vi "FileIO.vi"() -> ()   [LabVIEW 2012]
uses:
  <vilib>/Utility/file.llb/Write To Spreadsheet File (string).vi
  <vilib>/Utility/file.llb/Write To Spreadsheet File (DBL).vi
  <vilib>/Utility/file.llb/Read From Spreadsheet File (DBL).vi
panel:
  out "spreadsheet path":path
  out "Result":dbl[][](array[numeric]) format="%0.3f"
  out "Result":string
  out "text path":path
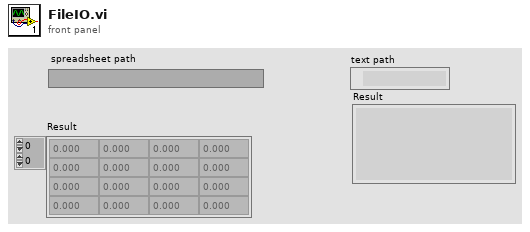
[diagram p1: front panel]
types:
  T1 = enum16{"open", "replace", "create", "open or create", "replace or create", "replace or create with confirmation"}
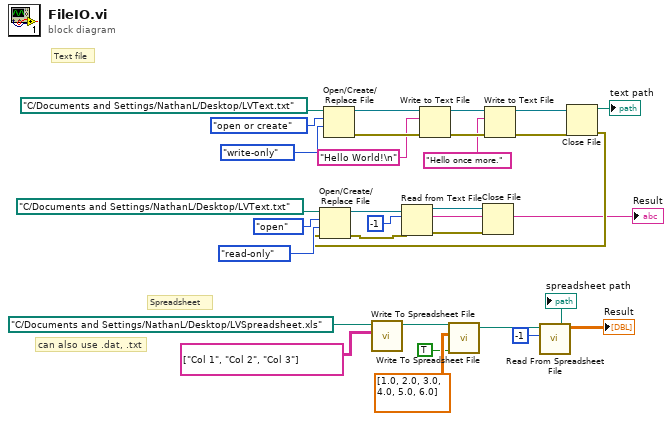
[diagram p0: block diagram]
diagram:
  # "can also use .dat, .txt"
  # "Spreadsheet"
  # "Text file"
  n1 = Open/Create/Replace File(file path (use dialog)=path "C:/Documents and Settings/NathanL/Desktop/LVText.txt", operation (0:open)=T1."open or create", access (0:read/write)=enum16{"read/write", "read-only", "write-only"}."write-only") -> (refnum out=w28:refnum<file>, error out=w26:errorcluster)  [unwired: 3 in, 1 out]
  n2 = call-poly <vilib>:"Write To Spreadsheet File.vi"("2D data"=string[][] [["Col 1", "Col 2", "Col 3"]] ("Array"), "file path (dialog if empty)"=path "C:/Documents and Settings/NathanL/Desktop/LVSpreadsheet.xls" ("file path (use dialog)")) -> ("new file path (Not A Path if cancelled)"=w4:path)  [unwired: 6 in]
  n3 = Write to Text File(file (use dialog)=w28, text="Hello World!\n", error in=w26) -> (refnum out=w27:refnum<file>, error out=w23:errorcluster)  [unwired: 1 in, 1 out]
  n4 = call-poly <vilib>:"Write To Spreadsheet File.vi"("append to file? (new file:F)"=TRUE, "2D data"=dbl[][] [[1.0, 2.0, 3.0], [4.0, 5.0, 6.0]], "file path (dialog if empty)"=w4) -> ("new file path (Not A Path if cancelled)"=w8:path)  [unwired: 5 in]
  n5 = Write to Text File(file (use dialog)=w27, text="Hello once more.", error in=w23) -> (refnum out=w24:refnum<file>, error out=w22:errorcluster)  [unwired: 1 in, 1 out]
  n6 = call-poly <vilib>:"Read From Spreadsheet File.vi"("number of rows (all:-1)"=-1, "file path (dialog if empty)"=w8) -> ("all rows"=→"Result":dbl[][], "new file path (Not A Path if cancelled)"=→"spreadsheet path":path)  [unwired: 5 in, 3 out]
  n7 = Close File(refnum=w24, error in=w22) -> (path=→"text path":path, error out=w17:errorcluster)
  n8 = Open/Create/Replace File(file path (use dialog)=path "C:/Documents and Settings/NathanL/Desktop/LVText.txt", error in=w17, operation (0:open)=T1."open", access (0:read/write)=enum16{"read/write", "read-only", "write-only"}."read-only") -> (refnum out=w16:refnum<file>, error out=w13:errorcluster)  [unwired: 2 in, 1 out]
  n9 = Read from Text File(file (use dialog)=w16, count=-1, error in=w13) -> (refnum out=w15:refnum<file>, text=→"Result":string, error out=w12:errorcluster)  [unwired: 1 in, 1 out]
  n10 = Close File(refnum=w15, error in=w12) -> ()  [unwired: 2 out]
